vi "Mux16.vi"(1 "B":bool[](array[boolean])=[FALSE, FALSE, FALSE, FALSE, FALSE, FALSE, FALSE, FALSE, FALSE, FALSE, FALSE, FALSE, FALSE, FALSE, FALSE, FALSE], 2 "A":bool[](array[boolean])=[FALSE, FALSE, FALSE, FALSE, FALSE, FALSE, FALSE, FALSE, FALSE, FALSE, FALSE, FALSE, FALSE, FALSE, FALSE, FALSE], 3 "s0":bool) -> (0 "z":bool[](array[boolean]))   [LabVIEW 2012]
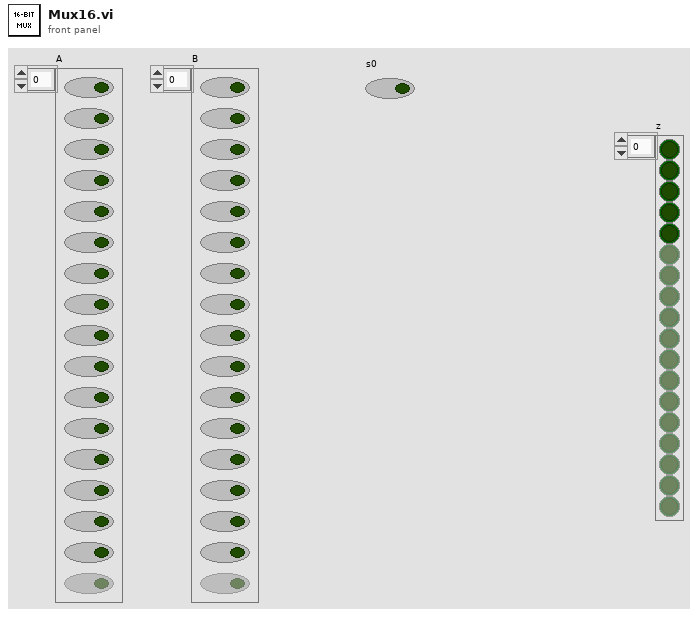
[diagram p1: front panel]
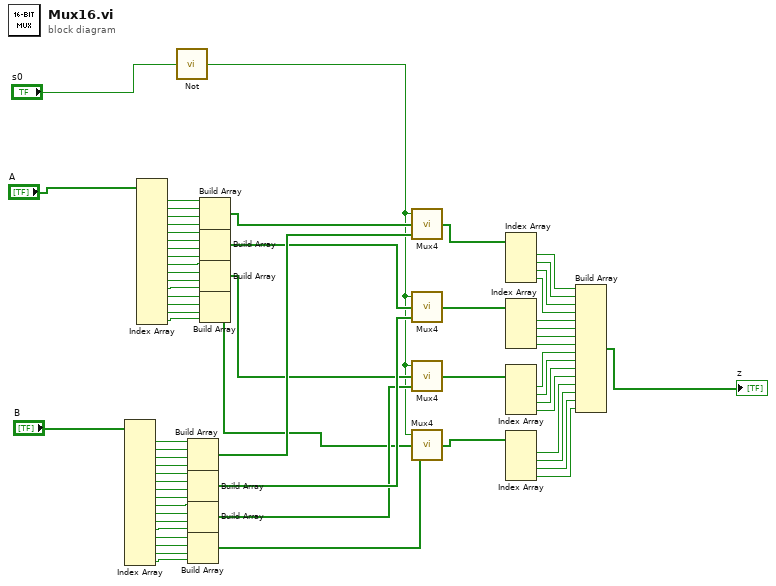
[diagram p0: block diagram]
diagram:
  n1 = Index Array(array="B") -> (element #1=w49:bool, element #2=w48:bool, element #3=w47:bool, element #4=w46:bool, element #5=w45:bool, element #6=w44:bool, element #7=w43:bool, element #8=w42:bool, element #9=w41:bool, element #10=w40:bool, element #11=w39:bool, element #12=w38:bool, element #13=w37:bool, element #14=w36:bool, element #15=w35:bool, element #16=w34:bool)  [unwired: 16 in]
  n2 = Index Array(array="A") -> (element #1=w65:bool, element #2=w64:bool, element #3=w63:bool, element #4=w62:bool, element #5=w61:bool, element #6=w60:bool, element #7=w59:bool, element #8=w58:bool, element #9=w57:bool, element #10=w56:bool, element #11=w55:bool, element #12=w54:bool, element #13=w53:bool, element #14=w52:bool, element #15=w51:bool, element #16=w50:bool)  [unwired: 16 in]
  n3 = call "Not.vi"("In"="s0") -> ("Out"=w1:bool)
  n4 = Build Array(w49, w48, w47, w46) -> (w30:bool[])
  n5 = Build Array(w45, w44, w43, w42) -> (w28:bool[])
  n6 = Build Array(w41, w40, w39, w38) -> (w27:bool[])
  n7 = Build Array(w37, w36, w35, w34) -> (w24:bool[])
  n8 = Build Array(w65, w64, w63, w62) -> (w31:bool[])
  n9 = Build Array(w61, w60, w59, w58) -> (w29:bool[])
  n10 = Build Array(w57, w56, w55, w54) -> (w26:bool[])
  n11 = Build Array(w53, w52, w51, w50) -> (w25:bool[])
  n12 = call "Mux4.vi"("B"=w30, "A"=w31, "s0"=w1) -> ("z"=w7:bool[])
  n13 = call "Mux4.vi"("B"=w28, "A"=w29, "s0"=w1) -> ("z"=w6:bool[])
  n14 = call "Mux4.vi"("B"=w27, "A"=w26, "s0"=w1) -> ("z"=w5:bool[])
  n15 = call "Mux4.vi"("B"=w24, "A"=w25, "s0"=w1) -> ("z"=w4:bool[])
  n16 = Index Array(array=w7) -> (element #1=w23:bool, element #2=w22:bool, element #3=w21:bool, element #4=w20:bool)  [unwired: 4 in]
  n17 = Index Array(array=w6) -> (element #1=w19:bool, element #2=w18:bool, element #3=w17:bool, element #4=w16:bool)  [unwired: 4 in]
  n18 = Index Array(array=w5) -> (element #1=w15:bool, element #2=w14:bool, element #3=w13:bool, element #4=w12:bool)  [unwired: 4 in]
  n19 = Index Array(array=w4) -> (element #1=w11:bool, element #2=w10:bool, element #3=w9:bool, element #4=w8:bool)  [unwired: 4 in]
  n20 = Build Array(w23, w22, w21, w20, w19, w18, w17, w16, w15, w14, w13, w12, w11, w10, w9, w8) -> (→"z":bool[])
